vi "SampleToJSON.vi"(8 "ErrorIn":errorcluster, 10 "Sample":T1, 11 "JSONIn":refnum<class "JSON Object.lvclass">) -> (0 "ErrorOut":errorcluster, 2 "JSONSamplePretty":string, 3 "JSONOut":refnum<class "JSON Object.lvclass">)   [LabVIEW 2016]
doc: "Convert Sample to JSON. Return also JSONOut to combine with other JSON objects."
uses:
  FallSensor/Sample.ctl
  FallSensor/Reading.ctl
  <vilib>/addons/JSON API/JSON Object/JSON Object.lvclass
  D:/Programy/National Instruments/LabVIEW 2016/vi.lib/addons/JSON API/JSON Value/JSON Value.lvclass
  <vilib>/addons/JSON API/JSON Object/Set Object Item by name.vi
  <vilib>/addons/JSON API/JSON Scalar/JSON Scalar.lvclass
  <vilib>/addons/JSON API/JSON Scalar/Set I32.vi
  <vilib>/addons/JSON API/JSON Value/Get as JSON string (pretty).vi
  <vilib>/addons/JSON API/Get Polymorphic/JSON GetSet.lvlib
  <vilib>/addons/JSON API/JSON Value/JSON Value.lvclass
panel:
  out "JSONSampleRaw":string
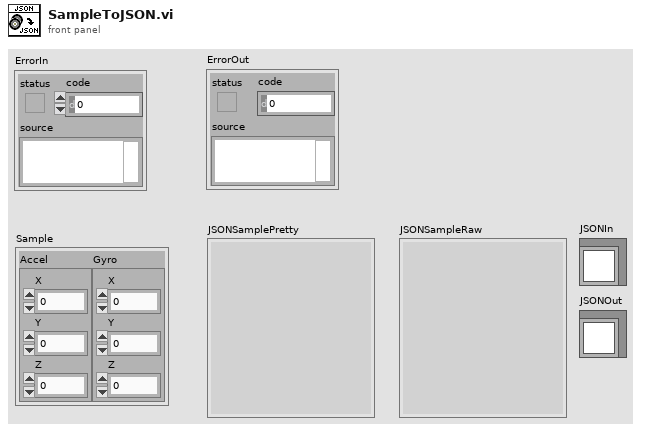
[diagram p1: front panel]
types:
  T1 = typedef "Sample.ctl" = cluster{"Accel":T2, "Gyro":T2}
  T2 = typedef "Reading.ctl" = cluster{"X":i16, "Y":i16, "Z":i16}
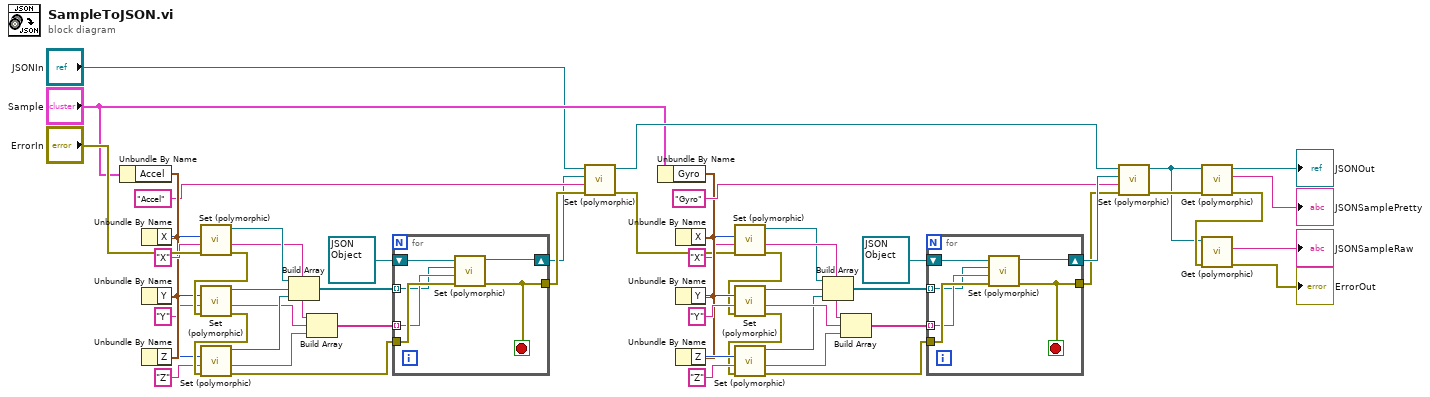
[diagram p0: block diagram]
diagram:
  n1 = Unbundle By Name("Sample") -> ("Accel"=w37:T2)
  n2 = Unbundle By Name(w37) -> ("X"=w38:i16)
  n3 = Unbundle By Name(w37) -> ("Y"=w35:i16)
  n4 = Unbundle By Name(w37) -> ("Z"=w33:i16)
  n5 = call-poly <vilib>:"Set (polymorphic).vi"("error in (no error)"="ErrorIn", "Numeric"=w38) -> ("error out"=w48:errorcluster, "JSON Scalar out"=w45:refnum<class "JSON Scalar.lvclass">)  [unwired: 8 in]
  n6 = call-poly <vilib>:"Set (polymorphic).vi"("error in (no error)"=w48, "Numeric"=w35) -> ("error out"=w47:errorcluster, "JSON Scalar out"=w46:refnum<class "JSON Scalar.lvclass">)  [unwired: 8 in]
  n7 = call-poly <vilib>:"Set (polymorphic).vi"("error in (no error)"=w47, "Numeric"=w33) -> ("error out"=w39:errorcluster, "JSON Scalar out"=w43:refnum<class "JSON Scalar.lvclass">)  [unwired: 8 in]
  n8 = Build Array(w45, w46, w43) -> (w41:refnum<class "JSON Scalar.lvclass">[])
  n9 = Build Array("X" ("name"), "Y" ("name"), "Z" ("name")) -> (w42:string[])
  n10 = for {
    tunnel: w42 -> [w52] mode=indexing
    tunnel: w41 -> [w51] mode=indexing
    tunnel: w39 -> [w53]
    shift-right: [w54] -> w30
    shift-left: refnum<class "JSON Object.lvclass"> refnum ("JSON Object out") -> [w55]
    tunnel: [w50] -> w31
    stop <- w50 stop-if-true
    n11 = call-poly <vilib>:"Set (polymorphic).vi"("error in (no error)"=w53, "name"=w52, "Value"=w51, "JSON Object in"=w55) -> ("error out"=w50:errorcluster, "JSON Object out"=w54:refnum<class "JSON Object.lvclass">)  [unwired: 5 in, 1 out]
  }
  n12 = call-poly <vilib>:"Set (polymorphic).vi"("error in (no error)"=w31, "name"="Accel", "Value"=w30, "JSON Object in"="JSONIn") -> ("error out"=w9:errorcluster, "JSON Object out"=w8:refnum<class "JSON Object.lvclass">)  [unwired: 5 in, 1 out]
  n13 = Unbundle By Name("Sample") -> ("Gyro"=w21:T2)
  n14 = Unbundle By Name(w21) -> ("X"=w20:i16)
  n15 = Unbundle By Name(w21) -> ("Y"=w23:i16)
  n16 = Unbundle By Name(w21) -> ("Z"=w25:i16)
  n17 = call-poly <vilib>:"Set (polymorphic).vi"("error in (no error)"=w9, "Numeric"=w20) -> ("error out"=w10:errorcluster, "JSON Scalar out"=w13:refnum<class "JSON Scalar.lvclass">)  [unwired: 8 in]
  n18 = call-poly <vilib>:"Set (polymorphic).vi"("error in (no error)"=w10, "Numeric"=w23) -> ("error out"=w11:errorcluster, "JSON Scalar out"=w12:refnum<class "JSON Scalar.lvclass">)  [unwired: 8 in]
  n19 = call-poly <vilib>:"Set (polymorphic).vi"("error in (no error)"=w11, "Numeric"=w25) -> ("error out"=w19:errorcluster, "JSON Scalar out"=w15:refnum<class "JSON Scalar.lvclass">)  [unwired: 8 in]
  n20 = Build Array(w13, w12, w15) -> (w17:refnum<class "JSON Scalar.lvclass">[])
  n21 = Build Array("X" ("name"), "Y" ("name"), "Z" ("name")) -> (w16:string[])
  n22 = for {
    tunnel: w16 -> [w58] mode=indexing
    tunnel: w17 -> [w57] mode=indexing
    tunnel: w19 -> [w59]
    shift-right: [w60] -> w28
    shift-left: refnum<class "JSON Object.lvclass"> refnum ("JSON Object out") -> [w61]
    tunnel: [w56] -> w27
    stop <- w56 stop-if-true
    n23 = call-poly <vilib>:"Set (polymorphic).vi"("error in (no error)"=w59, "name"=w58, "Value"=w57, "JSON Object in"=w61) -> ("error out"=w56:errorcluster, "JSON Object out"=w60:refnum<class "JSON Object.lvclass">)  [unwired: 5 in, 1 out]
  }
  n24 = call-poly <vilib>:"Set (polymorphic).vi"("error in (no error)"=w27, "name"="Gyro", "Value"=w28, "JSON Object in"=w8) -> ("error out"=w5:errorcluster, "JSON Object out"=w1:refnum<class "JSON Object.lvclass">)  [unwired: 5 in, 1 out]
  "JSONOut" <- w1
  n25 = call-poly <vilib>:"Get (polymorphic).vi"("error in (no error)"=w5, "JSON Value in"=w1) -> ("error out"=w4:errorcluster, "<JSON>"=→"JSONSamplePretty":string)  [unwired: 8 in]
  n26 = call-poly <vilib>:"Get (polymorphic).vi"("error in (no error)"=w4, "JSON Value in"=w1) -> ("error out"=→"ErrorOut":errorcluster, "<JSON>"=→"JSONSampleRaw":string)  [unwired: 8 in]
